vi "CalculateAmplitudeModulationWithBypass.vi"(8 "input valid":bool=TRUE, 10 "AM_factor":fxp<+/-,16,2>, 11 "Data in":fxp<+/-,32,14>[](array[numeric])=[0.0, 0.0, 0.0, 0.0]) -> (0 "output valid":bool, 3 "Data out":fxp<+/-,32,14>[](array[numeric]))   [LabVIEW 2018]
doc: "Calculates various combinations on I_in, Q_in and cos(fi) and sin(fi) to be used later to delay the output signal"
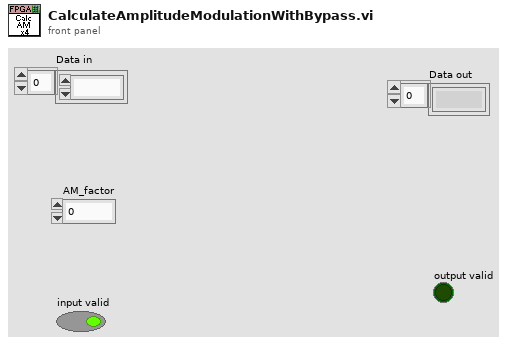
[diagram p1: front panel]
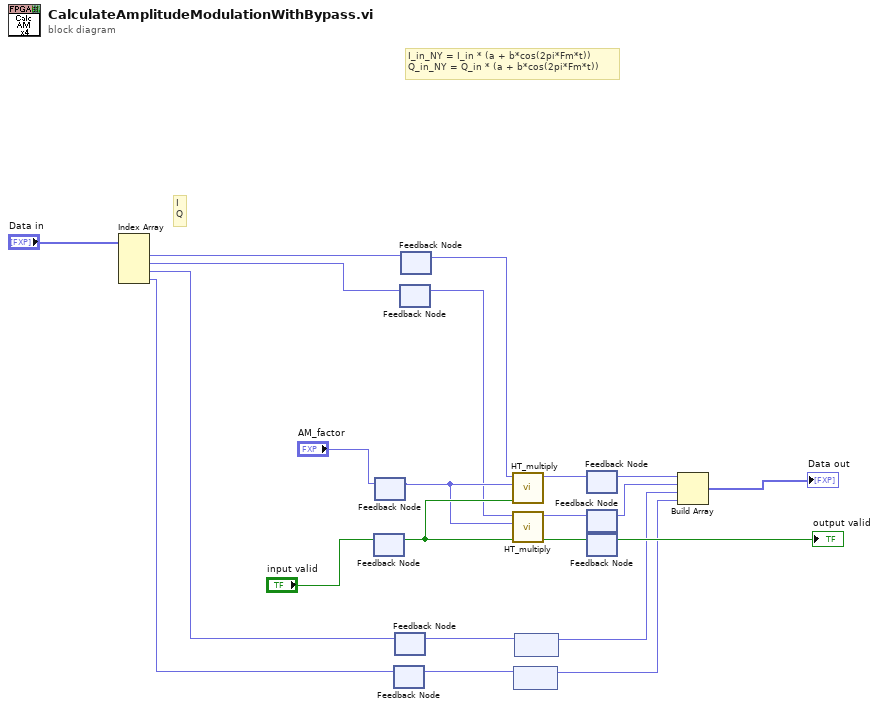
[diagram p0: block diagram]
diagram:
  # "I\nQ"
  # "I_in_NY = I_in * (a + b*cos(2pi*Fm*t))\nQ_in_NY = Q_in * (a + b*cos(2pi*Fm*t))"
  n1 = Index Array(array="Data in") -> (element #1=w10:fxp<+/-,32,14>, element #2=w8:fxp<+/-,32,14>, element #3=w6:fxp<+/-,32,14>, element #4=w5:fxp<+/-,32,14>)  [unwired: 4 in]
  n2 = feedback #1() -> (w13:bool)  [unwired: 1 in]
  n3 = feedback-in #1("input valid") -> ()
  n4 = feedback #2() -> (w11:fxp<+/-,16,2>)  [unwired: 1 in]
  n5 = feedback-in #2("AM_factor") -> ()
  n6 = feedback #3() -> (w3:fxp<+/-,32,14>)  [unwired: 1 in]
  n7 = feedback-in #3(w5) -> ()
  n8 = feedback #4() -> (w4:fxp<+/-,32,14>)  [unwired: 1 in]
  n9 = feedback-in #4(w6) -> ()
  n10 = feedback #5() -> (w7:fxp<+/-,32,14>)  [unwired: 1 in]
  n11 = feedback-in #5(w8) -> ()
  n12 = feedback #6() -> (w9:fxp<+/-,32,14>)  [unwired: 1 in]
  n13 = feedback-in #6(w10) -> ()
  n14 = call "HT_multiply.vi"("input valid"=w13, "y"=w11, "x"=w9) -> ("x*y"=w21:fxp<+/-,32,14>)  [unwired: 7 in, 1 out]
  n15 = call "HT_multiply.vi"("input valid"=w13, "y"=w11, "x"=w7) -> ("output valid"=w15:bool, "x*y"=w20:fxp<+/-,32,14>)  [unwired: 7 in]
  n16 = feedback #7() -> (w1:fxp<+/-,32,14>)  [unwired: 1 in]
  n17 = feedback-in #7(w3) -> ()
  n18 = feedback #8() -> (w2:fxp<+/-,32,14>)  [unwired: 1 in]
  n19 = feedback-in #8(w4) -> ()
  n20 = feedback #9() -> (w18:fxp<+/-,32,14>)  [unwired: 1 in]
  n21 = feedback-in #9(w21) -> ()
  n22 = feedback #10() -> (w17:fxp<+/-,32,14>)  [unwired: 1 in]
  n23 = feedback-in #10(w20) -> ()
  n24 = feedback #11() -> (→"output valid":bool)  [unwired: 1 in]
  n25 = feedback-in #11(w15) -> ()
  n26 = Build Array(w18, w17, w2, w1) -> (→"Data out":fxp<+/-,32,14>[])
